vi "main_control.vi"() -> ()   [LabVIEW 2018]
uses:
  Device VIs/Verbal.vi
panel:
  out "Motion":bool
  in  "单步时间ms":u32=100
  in  "CH2归0":bool
  in  "CH1归0":bool
  out "OK":bool
  in  "制动":bool
  in  "CH2启动":bool
  in  "CH1启动":bool
  in  "CH2 运动步数":i32
  in  "CH1 运动步数":i32
  out "CH2 当前位置":i32
  out "CH1 当前位置":i32
  out "状态":string
  out "error out":errorcluster
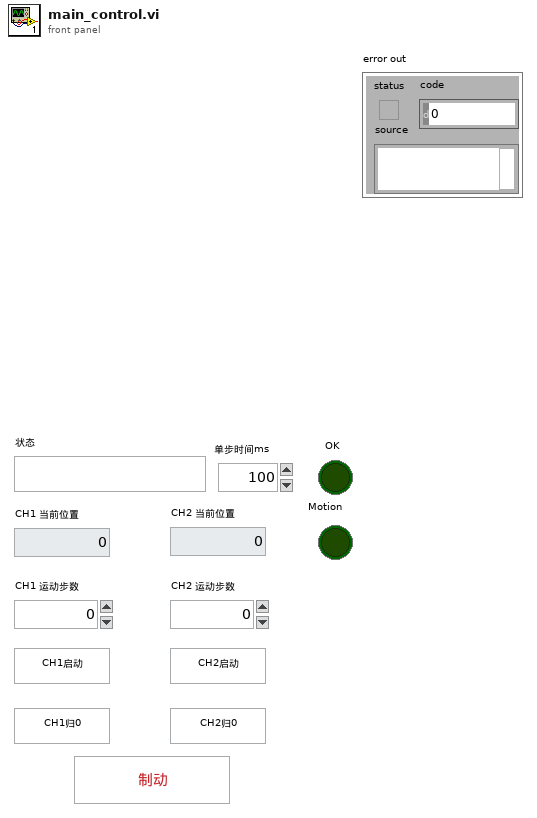
[diagram p1: front panel]
types:
  T1 = cluster{"DeviceKey":string, "Device Address":i32, "Controller Name":string}[]
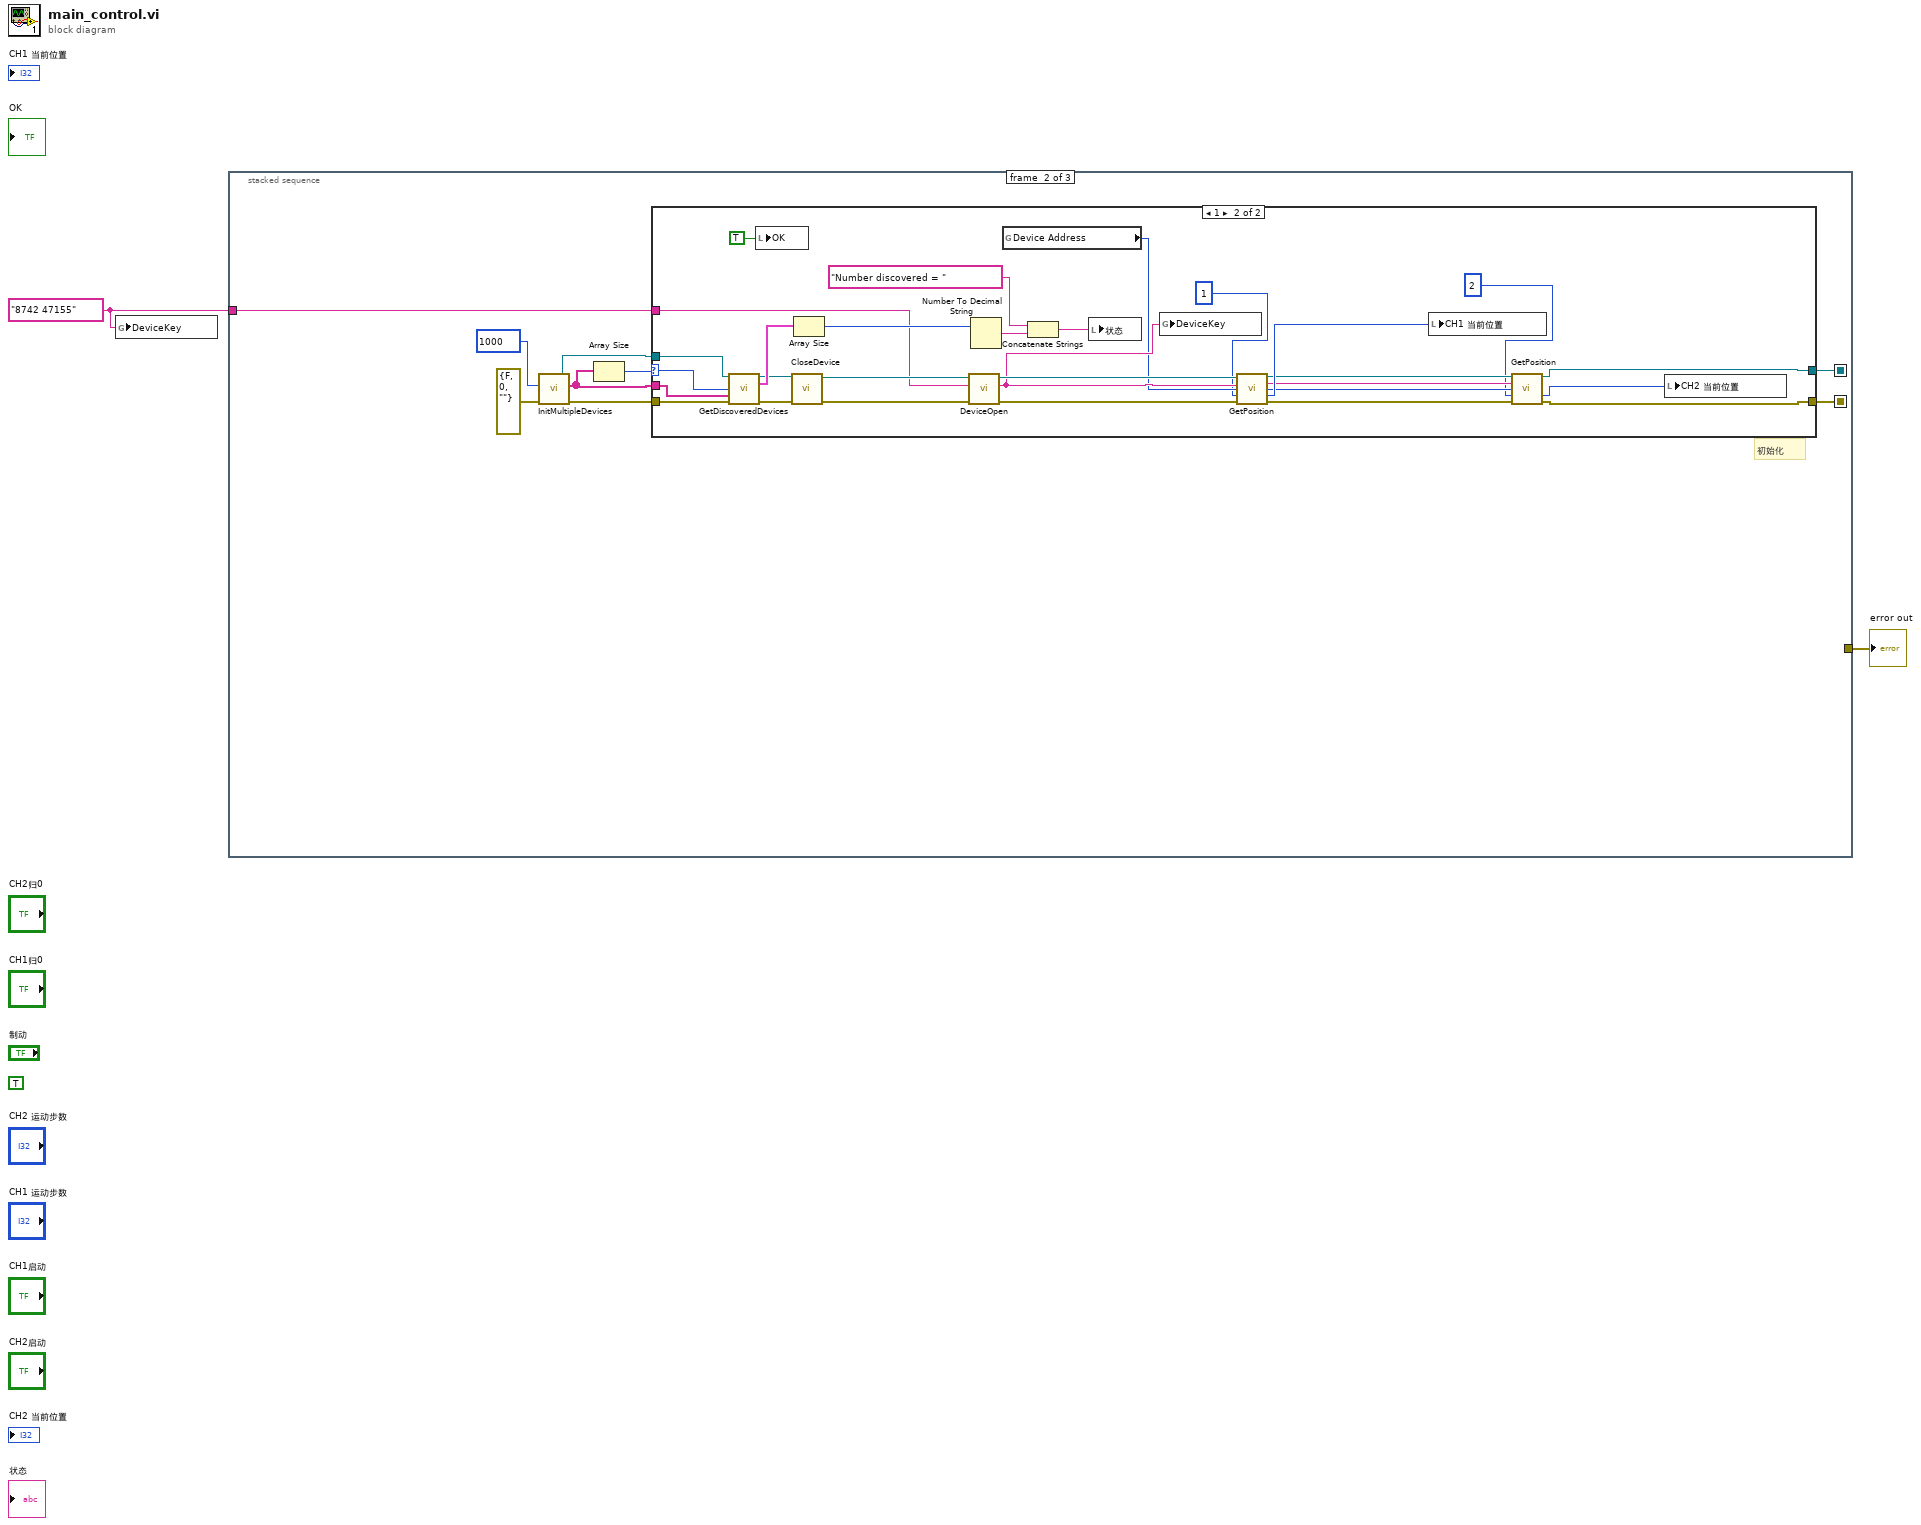
[diagram p0: block diagram]
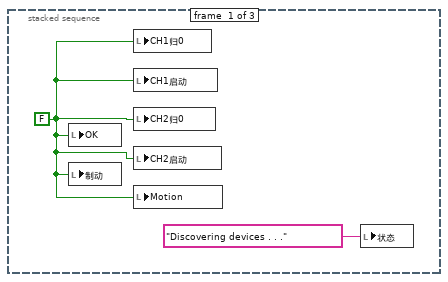
[diagram p2: hidden frame]
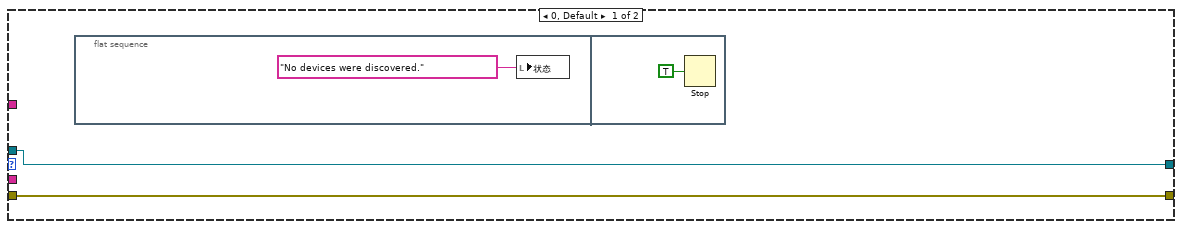
[diagram p3: hidden frame]
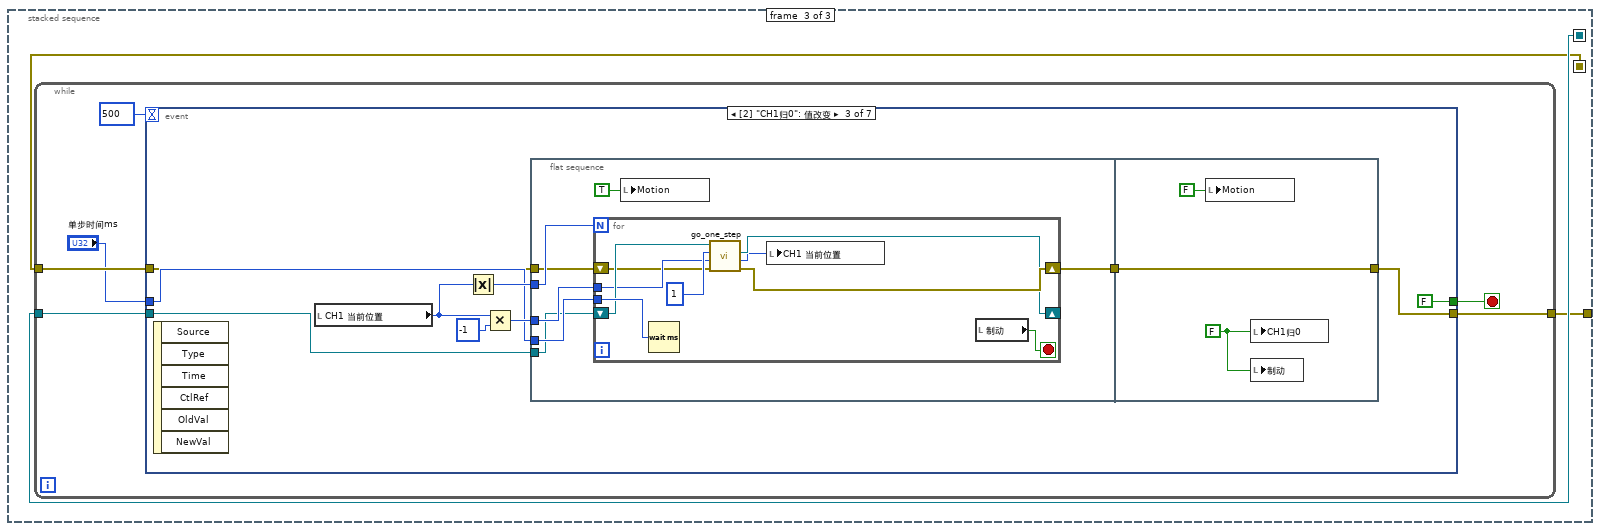
[diagram p4: hidden frame]
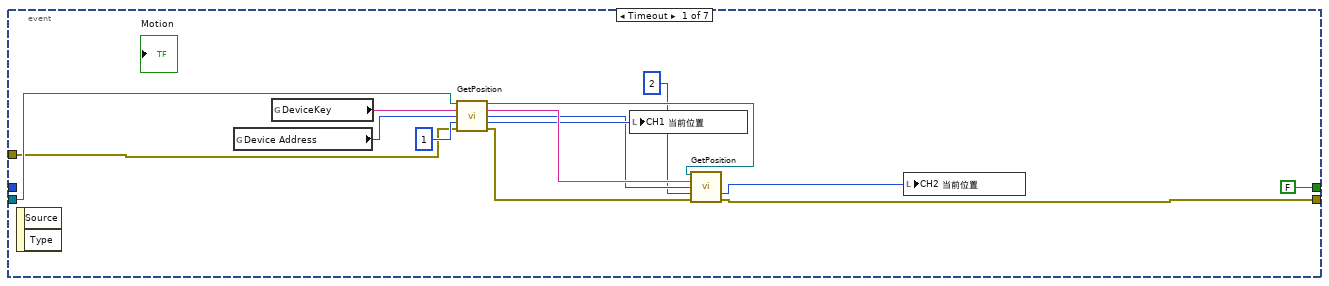
[diagram p5: hidden frame]
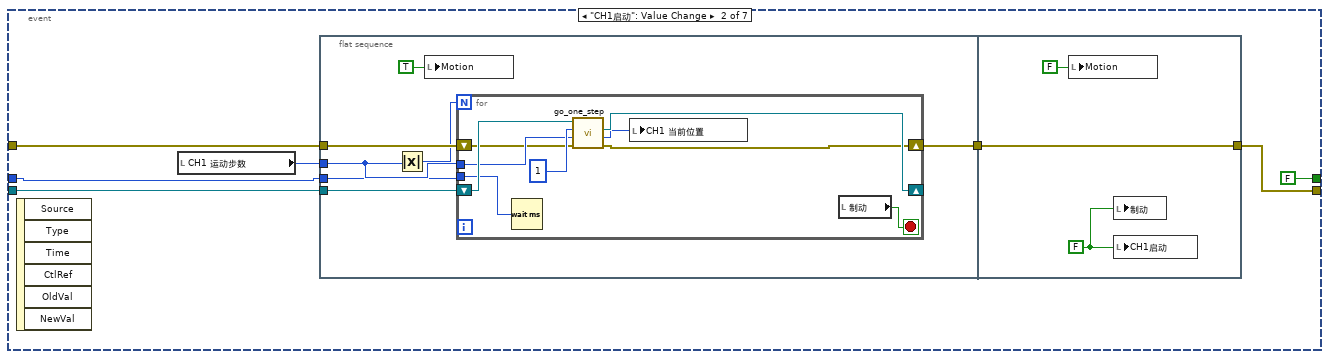
[diagram p6: hidden frame]
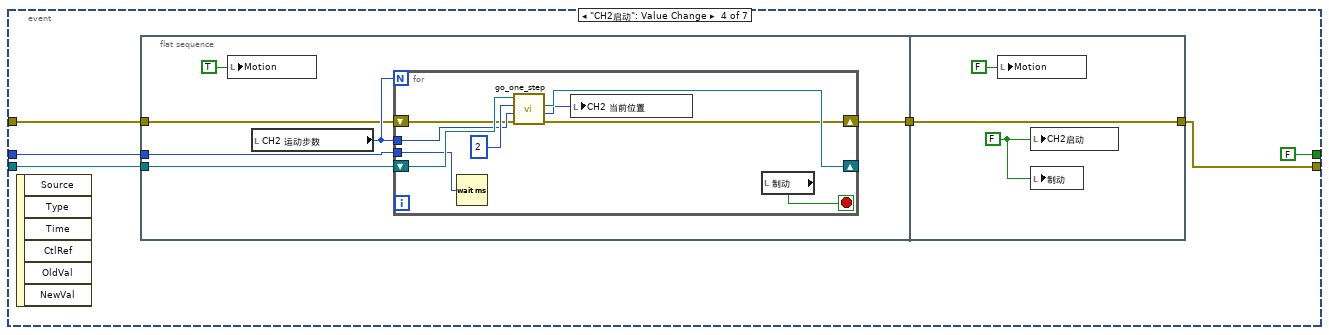
[diagram p7: hidden frame]
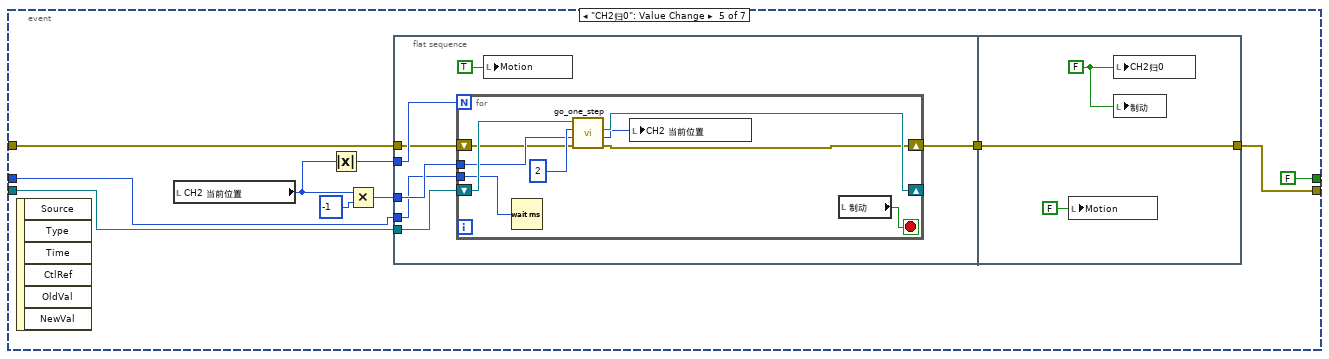
[diagram p8: hidden frame]
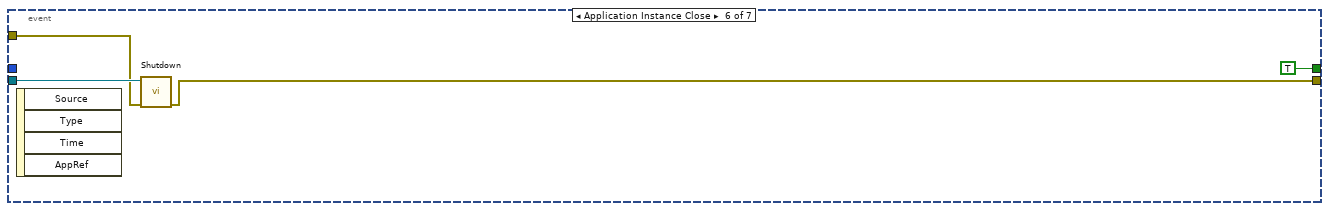
[diagram p9: hidden frame]
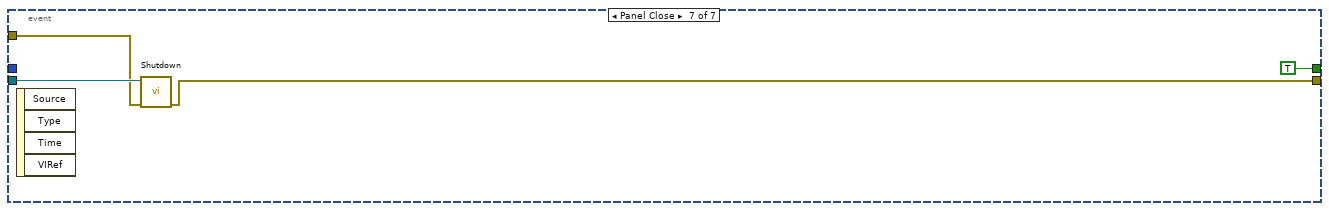
[diagram p10: hidden frame]
diagram:
  (unwired) TRUE
  w2 = "8742 47155" ("Message")
  n1 = global write "Verbal.vi" "DeviceKey"(w2) -> ()
  n2 = stacked-sequence {
    seq-local: [_ w6 _] -> [_ _ w49]
    seq-local: [_ w5 _] -> [_ _ w48]
    tunnel: w2 -> [_ w7 _]
    tunnel: [_ _ w47] -> w1
    frame #0 {
      w3 = FALSE ("Motion")
      n3 = local write "OK"(w3) -> ()
      n4 = local write "制动"(w3) -> ()
      n5 = local write "CH1归0"(w3) -> ()
      n6 = local write "CH1启动"(w3) -> ()
      n7 = local write "CH2归0"(w3) -> ()
      n8 = local write "CH2启动"(w3) -> ()
      n9 = local write "Motion"(w3) -> ()
      n10 = local write "状态"("Discovering devices . . ." ("Message")) -> ()
    }
    frame #1 {
      # "初始化"
      n11 = call "InitMultipleDevices.vi"("error in (no error)"=errorcluster {"status"=FALSE, "code"=0, "source"=""}, "msecDelayForDiscovery"=1000) -> ("error out"=w8:errorcluster, "DeviceKey List Out"=w9:string[], "CmdLib Out"=w10:refnum<k24>)  [unwired: 3 in]
      n12 = Array Size(array=w9) -> (size(s)=w11:i32)
      n13 = case shown="1" w11 {
        selector: w11 -> [_ w42]
        tunnel: w10 -> [w15 w43]
        tunnel: w9 -> [_ w41]
        tunnel: w8 -> [w14 w40]
        tunnel: w7 -> [_ w36]
        tunnel: [w15 w21] -> w6
        tunnel: [w14 w19] -> w5
        frame 0, Default {
          n14 = flat-sequence {
            frame #0 {
              n15 = local write "状态"("No devices were discovered." ("Input String")) -> ()
            }
            frame #1 {
              n16 = Stop(stop? (T)=TRUE ("停止？(T)")) -> ()
            }
          }
        }
        frame 1 {
          n17 = call "GetDiscoveredDevices.vi"("CmdLib In"=w43, "Master Count"=w42, "DeviceKey List"=w41, "error in"=w40) -> ("CmdLib Out"=w38:refnum<k24>, "Device Array"=w39:T1, "error out"=w35:errorcluster)  [unwired: 9 in]
          n18 = local write "OK"(TRUE ("等待指令")) -> ()
          n19 = call "CloseDevice.vi"("error in"=w35, "CmdLib In"=w38) -> ("error out"=w34:errorcluster, "CmdLib Out"=w37:refnum<k24>)  [unwired: 8 in]
          n20 = Array Size(array=w39) -> (size(s)=w46:i32)
          n21 = call "DeviceOpen.vi"("error in (no error)"=w34, "DeviceKey In"=w36, "CmdLib In"=w37) -> ("error out"=w29:errorcluster, "DeviceKey Out"=w32:string, "CmdLib Out"=w33:refnum<k24>)  [unwired: 2 in]
          n22 = Number To Decimal String(number=w46) -> (decimal integer string=w44:string)  [unwired: 1 in]
          n23 = global read "Verbal.vi" "Device Address"() -> (w31:i32)
          n24 = Concatenate Strings("Number discovered = " ("string"), w44) -> (w20:string)
          n25 = local write "状态"(w20) -> ()
          n26 = global write "Verbal.vi" "DeviceKey"(w32) -> ()
          n27 = call "GetPosition.vi"("CmdLib In"=w33, "DeviceKey In"=w32, "Device Address In"=w31, "Motor"=1, "error in (no error)"=w29) -> ("CmdLib Out"=w27:refnum<k24>, "DeviceKey Out"=w26:string, "Device Address Out"=w25:i32, "Position"=w28:i32, "error out"=w23:errorcluster)  [unwired: 6 in]
          n28 = local write "CH1 当前位置"(w28) -> ()
          n29 = call "GetPosition.vi"("CmdLib In"=w27, "DeviceKey In"=w26, "Device Address In"=w25, "Motor"=2, "error in (no error)"=w23) -> ("CmdLib Out"=w21:refnum<k24>, "Position"=w22:i32, "error out"=w19:errorcluster)  [unwired: 6 in, 2 out]
          n30 = local write "CH2 当前位置"(w22) -> ()
        }
      }
    }
    frame #2 {
      n31 = while {
        tunnel: w49 -> [w54]
        tunnel: w48 -> [w53]
        tunnel: [w52] -> w47
        stop <- w51 stop-if-true
        n32 = event shown="[2] \"CH1归0\": 值改变" {
          selector: _ -> [_ _ _ _ _ _ _]
          dyn-events: _ -> [_ _ _ _ _ _ _]
          timeout: 500 -> [_ _ _ _ _ _ _]
          tunnel: w54 -> [w69 w76 w100 w130 w154 w181 w185]
          tunnel: w53 -> [w58 w75 w99 w128 w153 w180 w184]
          tunnel: [w56 w74 w97 w129 w152 w179 w183] -> w52
          tunnel: [FALSE FALSE FALSE FALSE FALSE TRUE TRUE] -> w51
          tunnel: "单步时间ms" -> [_ w71 w101 w126 w150 _ _]
          event Timeout {
            n33 = event-data() -> ()  [unwired: 1 in, 2 out]
            n34 = global read "Verbal.vi" "Device Address"() -> (w67:i32)
            n35 = global read "Verbal.vi" "DeviceKey"() -> (w68:string)
            n36 = call "GetPosition.vi"("CmdLib In"=w69, "DeviceKey In"=w68, "Device Address In"=w67, "Motor"=1, "error in (no error)"=w58) -> ("CmdLib Out"=w65:refnum<k24>, "DeviceKey Out"=w64:string, "Device Address Out"=w62:i32, "Position"=w63:i32, "error out"=w57:errorcluster)  [unwired: 6 in]
            n37 = local write "CH1 当前位置"(w63) -> ()
            n38 = call "GetPosition.vi"("CmdLib In"=w65, "DeviceKey In"=w64, "Device Address In"=w62, "Motor"=2, "error in (no error)"=w57) -> ("Position"=w60:i32, "error out"=w56:errorcluster)  [unwired: 6 in, 3 out]
            n39 = local write "CH2 当前位置"(w60) -> ()
          }
          event "CH1启动": Value Change {
            n40 = event-data() -> ()  [unwired: 1 in, 6 out]
            n41 = local read "CH1 运动步数"() -> (w72:i32)
            n42 = flat-sequence {
              tunnel: w76 -> [w83]
              tunnel: w75 -> [w82]
              tunnel: w72 -> [w79]
              tunnel: w71 -> [w78]
              tunnel: [w81] -> w70
              tunnel: [w95] -> w74
              tunnel: w70 -> [w95]
              frame #0 {
                n43 = Absolute Value(x=w79) -> (abs(x)=w80:i32)
                n44 = local write "Motion"(TRUE ("Motion")) -> ()
                n45 = for {
                  N: w80 -> [_]
                  shift-right: [w86] -> w81
                  shift-left: w82 -> [w88]
                  shift-right: [w91] -> _
                  shift-left: w83 -> [w92]
                  tunnel: w79 -> [w89]
                  tunnel: w78 -> [w85]
                  stop <- w84 stop-if-true
                  n46 = Wait (ms)(milliseconds to wait=w85) -> ()  [unwired: 1 out]
                  n47 = call "go_one_step.vi"("error in"=w88, "Step"=w89, "Motor"=1, "CmdLib In"=w92) -> ("error out"=w86:errorcluster, "Position"=w87:i32, "CmdLib Out"=w91:refnum<k24>)  [unwired: 1 in]
                  n48 = local write "CH1 当前位置"(w87) -> ()
                  n49 = local read "制动"() -> (w84:bool)
                }
              }
              frame #1 {
                w94 = FALSE ("制动")
                n50 = local write "Motion"(FALSE ("Motion")) -> ()
                n51 = local write "制动"(w94) -> ()
                n52 = local write "CH1启动"(w94) -> ()
              }
            }
          }
          event "CH1归0": Value Change {
            n53 = event-data() -> ()  [unwired: 1 in, 6 out]
            n54 = local read "CH1 当前位置"() -> (w104:i32)
            n55 = Absolute Value(x=w104) -> (abs(x)=w105:i32)
            n56 = Multiply(x=w104, y=-1) -> (x*y=w102:i32)
            n57 = flat-sequence {
              tunnel: w105 -> [w112]
              tunnel: w102 -> [w111]
              tunnel: w101 -> [w110]
              tunnel: w100 -> [w109]
              tunnel: w99 -> [w108]
              tunnel: [w107] -> w96
              tunnel: [w124] -> w97
              tunnel: w96 -> [w124]
              frame #0 {
                n58 = for {
                  N: w112 -> [_]
                  tunnel: w111 -> [w118]
                  tunnel: w110 -> [w121]
                  shift-right: [w116] -> w107
                  shift-left: w108 -> [w117]
                  shift-right: [w115] -> _
                  shift-left: w109 -> [w120]
                  stop <- w113 stop-if-true
                  n59 = Wait (ms)(milliseconds to wait=w121) -> ()  [unwired: 1 out]
                  n60 = call "go_one_step.vi"("error in"=w117, "Step"=w118, "Motor"=1, "CmdLib In"=w120) -> ("error out"=w116:errorcluster, "Position"=w114:i32, "CmdLib Out"=w115:refnum<k24>)  [unwired: 1 in]
                  n61 = local write "CH1 当前位置"(w114) -> ()
                  n62 = local read "制动"() -> (w113:bool)
                }
                n63 = local write "Motion"(TRUE ("Motion")) -> ()
              }
              frame #1 {
                w123 = FALSE ("制动")
                n64 = local write "Motion"(FALSE ("Motion")) -> ()
                n65 = local write "CH1归0"(w123) -> ()
                n66 = local write "制动"(w123) -> ()
              }
            }
          }
          event "CH2启动": Value Change {
            n67 = event-data() -> ()  [unwired: 1 in, 6 out]
            n68 = flat-sequence {
              tunnel: w130 -> [w136]
              tunnel: w128 -> [w133]
              tunnel: w126 -> [w132]
              tunnel: [w134] -> w125
              tunnel: [w148] -> w129
              tunnel: w125 -> [w148]
              frame #0 {
                n69 = local write "Motion"(TRUE ("Motion")) -> ()
                n70 = local read "CH2 运动步数"() -> (w135:i32)
                n71 = for {
                  N: w135 -> [_]
                  tunnel: w135 -> [w143]
                  shift-right: [w142] -> _
                  shift-left: w136 -> [w145]
                  shift-right: [w140] -> w134
                  shift-left: w133 -> [w139]
                  tunnel: w132 -> [w138]
                  stop <- w137 stop-if-true
                  n72 = Wait (ms)(milliseconds to wait=w138) -> ()  [unwired: 1 out]
                  n73 = call "go_one_step.vi"("error in"=w139, "Step"=w143, "Motor"=2, "CmdLib In"=w145) -> ("error out"=w140:errorcluster, "Position"=w141:i32, "CmdLib Out"=w142:refnum<k24>)  [unwired: 1 in]
                  n74 = local write "CH2 当前位置"(w141) -> ()
                  n75 = local read "制动"() -> (w137:bool)
                }
              }
              frame #1 {
                w147 = FALSE
                n76 = local write "Motion"(FALSE ("Motion")) -> ()
                n77 = local write "CH2启动"(w147) -> ()
                n78 = local write "制动"(w147) -> ()
              }
            }
          }
          event "CH2归0": Value Change {
            n79 = event-data() -> ()  [unwired: 1 in, 6 out]
            n80 = local read "CH2 当前位置"() -> (w157:i32)
            n81 = Absolute Value(x=w157) -> (abs(x)=w158:i32)
            n82 = Multiply(x=w157, y=-1) -> (x*y=w155:i32)
            n83 = flat-sequence {
              tunnel: w158 -> [w165]
              tunnel: w155 -> [w164]
              tunnel: w154 -> [w163]
              tunnel: w153 -> [w162]
              tunnel: w150 -> [w160]
              tunnel: [w161] -> w149
              tunnel: [w177] -> w152
              tunnel: w149 -> [w177]
              frame #0 {
                n84 = for {
                  N: w165 -> [_]
                  tunnel: w164 -> [w171]
                  shift-right: [w173] -> _
                  shift-left: w163 -> [w174]
                  shift-right: [w169] -> w161
                  shift-left: w162 -> [w170]
                  tunnel: w160 -> [w167]
                  stop <- w166 stop-if-true
                  n85 = Wait (ms)(milliseconds to wait=w167) -> ()  [unwired: 1 out]
                  n86 = call "go_one_step.vi"("error in"=w170, "Step"=w171, "Motor"=2, "CmdLib In"=w174) -> ("error out"=w169:errorcluster, "Position"=w168:i32, "CmdLib Out"=w173:refnum<k24>)  [unwired: 1 in]
                  n87 = local write "CH2 当前位置"(w168) -> ()
                  n88 = local read "制动"() -> (w166:bool)
                }
                n89 = local write "Motion"(TRUE ("Motion")) -> ()
              }
              frame #1 {
                w176 = FALSE ("制动")
                n90 = local write "Motion"(FALSE ("Motion")) -> ()
                n91 = local write "CH2归0"(w176) -> ()
                n92 = local write "制动"(w176) -> ()
              }
            }
          }
          event Application Instance Close {
            n93 = event-data() -> ()  [unwired: 1 in, 4 out]
            n94 = call "Shutdown.vi"("error in (no error)"=w180, "CmdLib In"=w181) -> ("error out"=w179:errorcluster)  [unwired: 4 in, 1 out]
          }
          event Panel Close {
            n95 = event-data() -> ()  [unwired: 1 in, 4 out]
            n96 = call "Shutdown.vi"("error in (no error)"=w184, "CmdLib In"=w185) -> ("error out"=w183:errorcluster)  [unwired: 4 in, 1 out]
          }
        }
      }
    }
  }
  "error out" <- w1
